vi "testMatrixGen.vi"() -> ()   [LabVIEW 2017]
panel:
  out "Intensity Graph":i32[][](graph)
  in  "index (page)":i32
  in  "Array":dbl[](array[numeric])
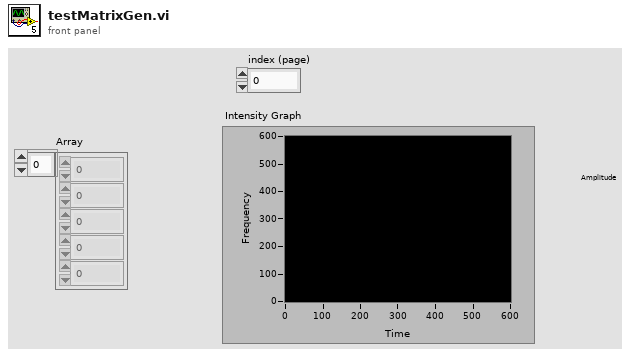
[diagram p1: front panel]
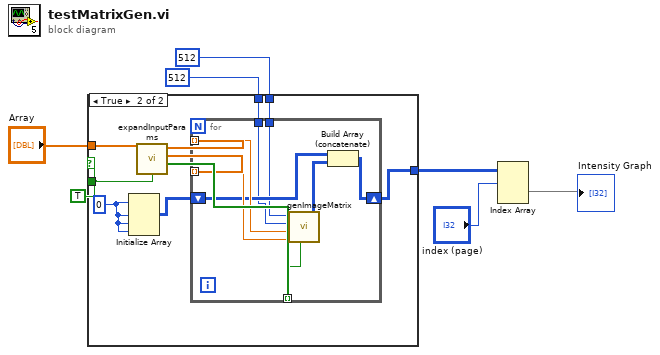
[diagram p0: block diagram]
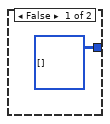
[diagram p2: hidden frame]
diagram:
  w4 = TRUE
  n1 = case shown="True" w4 {
    tunnel: 512 ("X Resolution") -> [_ w15]
    tunnel: 512 ("Y resolution") -> [_ w14]
    tunnel: "Array" -> [_ w13]
    tunnel: w4 -> [_ w12]
    tunnel: [u8[][][] [] w11] -> w3
    frame False {
    }
    frame True {
      w9 = 0
      n2 = Initialize Array(w9, w9, w9, w9) -> (w10:i32[][][])
      n3 = call "expandInputParams.vi"("Profilometry?"=w12, "Frequencies"=w13) -> ("Orientation Vector"=w18:bool[], "Phase Vector"=w17:dbl[], "Frequency Vector"=w16:dbl[])  [unwired: 6 in, 1 out]
      n4 = for {
        tunnel: w18 -> [w26] mode=indexing
        tunnel: w17 -> [w25] mode=indexing
        tunnel: w16 -> [w24] mode=indexing
        shift-right: [w22] -> w11
        shift-left: w10 -> [w21]
        tunnel: w15 -> [w20]
        tunnel: w14 -> [w19]
        n5 = call "genImageMatrix.vi"("Orientation"=w26, "Phase"=w25, "Cycles"=w24, "Y resolution"=w19, "X Resolution"=w20) -> ("Scan Image"=w23:u8[][])  [unwired: 5 in, 1 out]
        n6 = Build Array (concatenate)(w21, w23) -> (w22:i32[][][])
      }
    }
  }
  n7 = Index Array(array=w3, index (dim 0)="index (page)") -> (element=→"Intensity Graph":i32[][])  [unwired: 2 in]
